vi "Object_Get Attributes.vi"(8 "error in (no error)":errorcluster, 10 "Only Get DVR":bool, 11 "Object In":refnum<class "Object.lvclass">) -> (0 "error out":errorcluster, 1 "DataRef":refnum<data-value>, 2 "Data":T1, 3 "Object Out":refnum<class "Object.lvclass">)   [LabVIEW 2015, in "Front Panel Publisher.lvlib" / "Object.lvclass"]
uses:
  Object.lvclass
  Attributes.ctl
  Coordinates.ctl
  Object.lvclass/Object.ctl
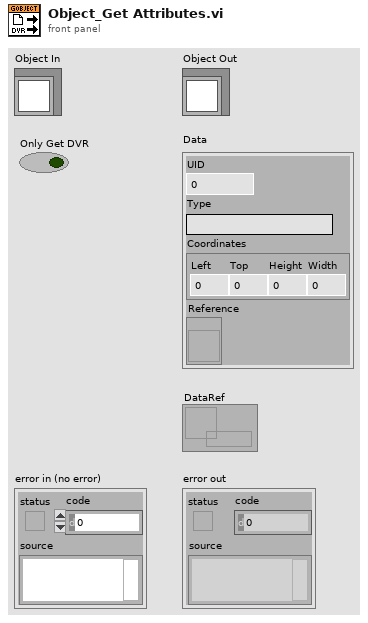
[diagram p1: front panel]
types:
  T1 = typedef "Front Panel Publisher.lvlib/Object.lvclass/Attributes.ctl" = cluster{"UID":i32, "Type":string, "Coordinates":T2, "Reference":refnum<vi>}
  T2 = typedef "Front Panel Publisher.lvlib/Object.lvclass/Coordinates.ctl" = cluster{"Left":i32, "Top":i32, "Height":u32, "Width":u32}
  T3 = typedef "FrontPanelPublisher.lvlib/Object.lvclass/Attributes.ctl" = cluster{"UID":i32, "Type":string, "Coordinates":T4, "Reference":refnum<vi>}
  T4 = typedef "FrontPanelPublisher.lvlib/Object.lvclass/Coordinates.ctl" = cluster{"Left":i32, "Top":i32, "Height":u32, "Width":u32}
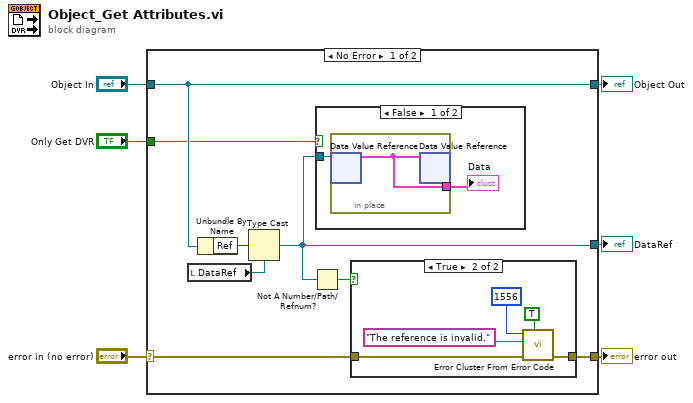
[diagram p0: block diagram]
diagram:
  n1 = case shown="No Error" "error in (no error)" {
    selector: "error in (no error)" -> [w9 w24]
    tunnel: [w7 w24] -> w5
    tunnel: [w14 w25] -> w3
    tunnel: "Object In" -> [w14 w25]
    tunnel: [w10 _] -> w2
    tunnel: "Only Get DVR" -> [w11 _]
    frame No Error {
      n2 = local read "DataRef"() -> (w12:refnum<data-value>)
      n3 = Unbundle By Name(w14) -> ("Ref"=w13:u32)
      n4 = Type Cast(type=w12, x=w13) -> (*(type *) &x=w10:refnum<data-value>)
      n5 = Not A Number/Path/Refnum?(number/path/refnum=w10) -> (NaN/Path/Refnum?=w8:bool)
      n6 = case shown="False" w11 {
        tunnel: w10 -> [w22 _]
        frame False {
          n7 = in-place {
            in-place-border: [w23] -> w21
            n8 = in-place-dvr #1(w22) -> (w23:T3)  [unwired: 1 out]
            n9 = in-place-dvr #1(w23) -> ()  [unwired: 2 out]
          }
          "Data" <- w21
        }
        frame True {
        }
      }
      n10 = case shown="True" w8 {
        tunnel: w9 -> [w15 w17]
        tunnel: [w15 w16] -> w7
        frame False {
        }
        frame True {
          n11 = call <vilib>:"Error Cluster From Error Code.vi"("show call chain? (False)"=TRUE, "error in (no error)"=w17, "error message (\"\")"="The reference is invalid." ("source"), "error code (0)"=1556 ("code")) -> ("error out"=w16:errorcluster)  [unwired: 5 in]
        }
      }
    }
    frame Error {
    }
  }
  "error out" <- w5
  "Object Out" <- w3
  "DataRef" <- w2
